vi "Global Parameters.vi"() -> ()   [LabVIEW 2020]
panel:
  in  "Tab Control":T1(tab)
  in  "Counter":tag="Dev1/ctr0"
  in  "Clock  Terminal":tag="/Dev1/PFI2"
  in  "Clock Frequency":dbl=50.0 format="%.6f"
  in  "Duty Cycle":dbl=0.5 format="%.6f"
  out "Scanner error":errorcluster
  out "Current Position(Global)":dbl[](array[numeric])
  # "After change the settings, please restart the clock to let the change effective."
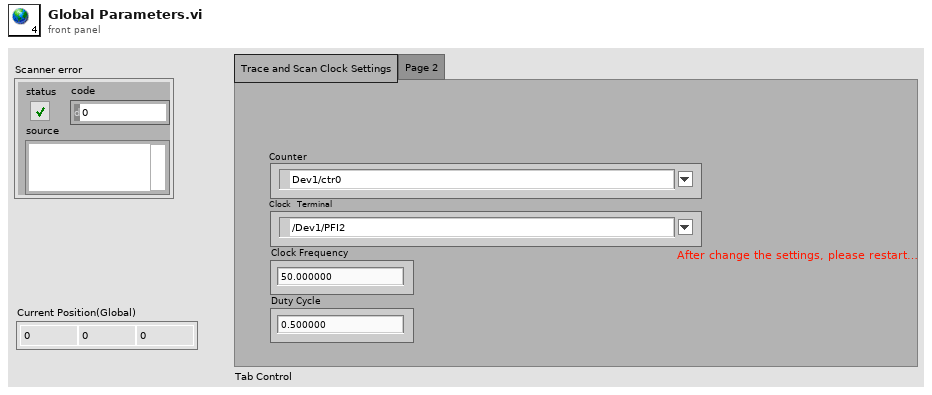
[diagram p1: front panel]
types:
  T1 = enum32{"Trace and Scan Clock Settings", "Page 2"}
diagram:
